vi "UDPListenFGV.vi"(8 "error in (no error)":errorcluster, 10 "Write Data":string, 11 "Enum":T1=enum."Write") -> (0 "error out":errorcluster, 3 "Read Data":string)   [LabVIEW 2017]
uses:
  TypeDefs/UDPListenFGVCtrl.ctl
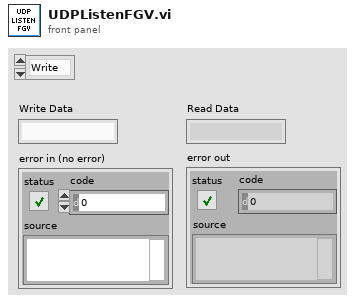
[diagram p1: front panel]
types:
  T1 = typedef "UDPListenFGVCtrl.ctl" = enum16{"Read", "Write"}
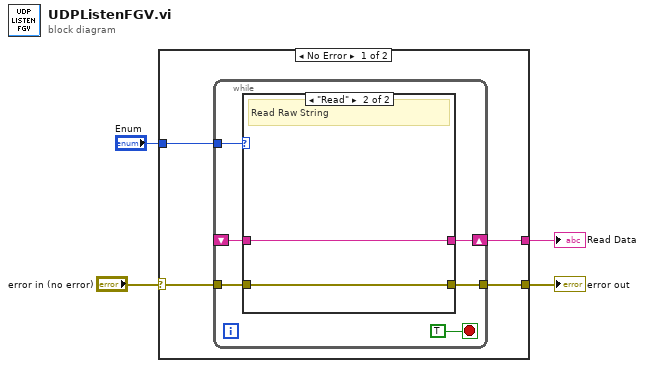
[diagram p0: block diagram]
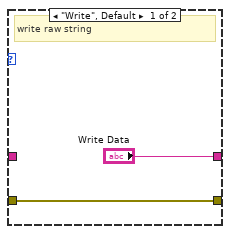
[diagram p2: hidden frame]
diagram:
  n1 = case shown="No Error" "error in (no error)" {
    selector: "error in (no error)" -> [w7 w19]
    tunnel: [w6 w19] -> w3
    tunnel: "Enum" -> [w8 _]
    tunnel: [w5 _] -> w2
    frame No Error {
      n2 = while {
        tunnel: w8 -> [w13]
        tunnel: w7 -> [w12]
        tunnel: [w11] -> w6
        shift-right: [w10] -> w5
        shift-left: _ -> [w9]
        stop <- TRUE stop-if-true
        n3 = case shown="\"Read\"" w13 {
          tunnel: w12 -> [w16 w18]
          tunnel: [w16 w18] -> w11
          tunnel: ["Write Data" w17] -> w10
          tunnel: w9 -> [_ w17]
          frame "Write", Default {
            # "write raw string"
          }
          frame "Read" {
            # "Read Raw String"
          }
        }
      }
    }
    frame Error {
    }
  }
  "error out" <- w3
  "Read Data" <- w2
